vi "TODO2_counter.vi"() -> ()   [LabVIEW 2020]
panel:
  in  "stop":bool
  in  "Reset":bool
  in  "counter by 2":bool
  in  "counter by 1":bool
  out "led 3":bool
  out "led 2":bool
  out "led 1":bool
  out "led 0":bool
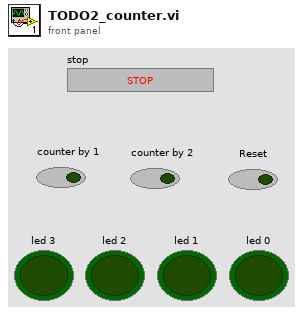
[diagram p1: front panel]
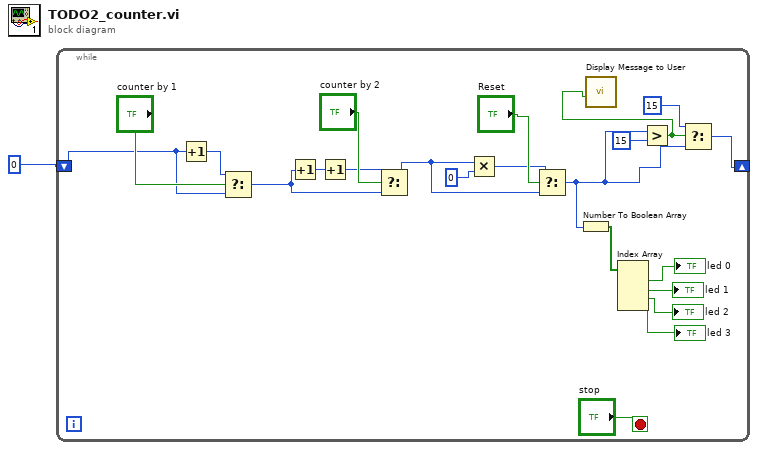
[diagram p0: block diagram]
diagram:
  n1 = while {
    shift-right: [w3] -> _
    shift-left: 0 -> [w20]
    stop <- "stop" stop-if-true
    n2 = Increment(x=w20) -> (x+1=w21:i32)
    n3 = Select(t=w21, s="counter by 1", f=w20) -> (s? t:f=w16:i32)
    n4 = Increment(x=w16) -> (x+1=w18:i32)
    n5 = Increment(x=w18) -> (x+1=w17:i32)
    n6 = Select(t=w17, s="counter by 2", f=w16) -> (s? t:f=w12:i32)
    n7 = Multiply(x=w12, y=0) -> (x*y=w13:i32)
    n8 = Select(t=w13, s="Reset", f=w12) -> (s? t:f=w4:i32)
    n9 = Number To Boolean Array(number=w4) -> (Boolean array=w11:bool[])
    n10 = Index Array(array=w11) -> (element #1=→"led 0":bool, element #2=→"led 1":bool, element #3=→"led 2":bool, element #4=→"led 3":bool)  [unwired: 4 in]
    n11 = Greater?(x=w4, y=15) -> (0:w2:bool)
    n12 = call "Display Message to User"("Enable"=w2) -> ()  [unwired: 9 in, 2 out]
    n13 = Select(t=15 ("y"), s=w2, f=w4) -> (s? t:f=w3:i32)
  }
